vi "Read Max.vi"(8 "error in (no error)":errorcluster, 11 "Measurement2D in":refnum<class "Measurement2D.lvclass">) -> (0 "error out":errorcluster, 2 "Max":dbl, 3 "Measurement2D out":refnum<class "Measurement2D.lvclass">)   [LabVIEW 2018, in "Measurement2D.lvclass"]
uses:
  Measurement2D.lvclass
  Measurement2D.lvclass/Measurement2D.ctl
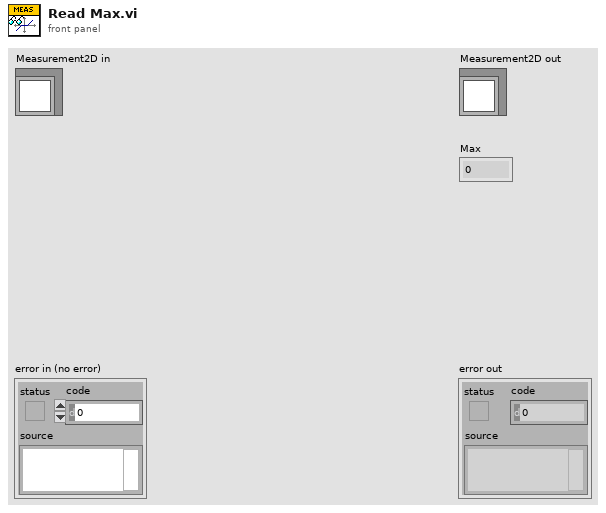
[diagram p1: front panel]
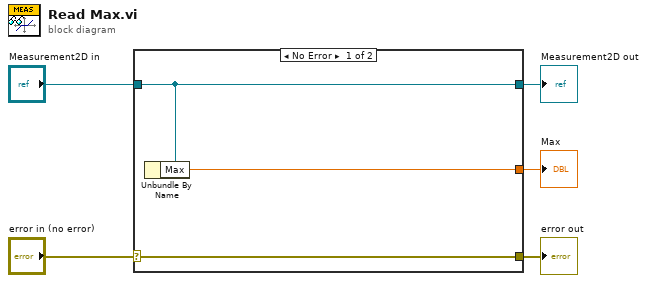
[diagram p0: block diagram]
diagram:
  n1 = case shown="No Error" "error in (no error)" {
    selector: "error in (no error)" -> [w8 w9]
    tunnel: [w8 w9] -> w4
    tunnel: [w7 w10] -> w2
    tunnel: "Measurement2D in" -> [w7 w10]
    tunnel: [w6 _] -> w1
    frame No Error {
      n2 = Unbundle By Name(w7) -> ("Max"=w6:dbl)
    }
    frame Error {
    }
  }
  "error out" <- w4
  "Measurement2D out" <- w2
  "Max" <- w1
